vi "Message Log ID to String.vi"(11 "Message Log ID":T1) -> (3 "Message Log ID String":string)   [LabVIEW 2017]
uses:
  Message Log ID.ctl
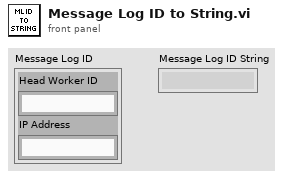
[diagram p1: front panel]
types:
  T1 = typedef "Message Log ID.ctl" = cluster{"Head Worker ID":string, "IP Address":string}
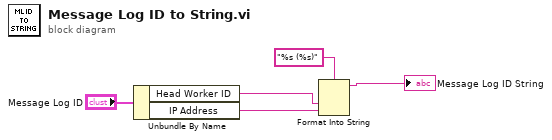
[diagram p0: block diagram]
diagram:
  n1 = Unbundle By Name("Message Log ID") -> ("Head Worker ID"=w2:string, "IP Address"=w1:string)
  n2 = Format Into String(format string="%s (%s)", w2, w1) -> (resulting string=→"Message Log ID String":string)  [unwired: 2 in, 1 out]
